vi "Sondenmodell.WriteZustandsgrössen.vi"(8 "Error in":errorcluster, 9 "Rücklauftemperatur Solekreislauf [°C]":dbl, 10 "Erdtemperatur [°C]":dbl, 11 "Sondemodell in":refnum<data-value>) -> (0 "Error out":errorcluster)   [LabVIEW 2016, in "Sondenmodell.lvclass"]
uses:
  Sondenmodell.lvclass
  Sondenmodell.lvclass/Sondenmodell.ctl
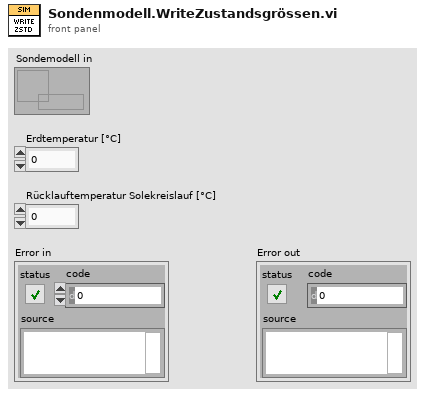
[diagram p1: front panel]
types:
  T1 = typedef "Sondenmodell.lvclass/Sondenmodell.Zustandsgrössen.ctl" = cluster{"Erdtemperatur [°C]":dbl, "Rücklauftemperatur Solekreislauf [°C]":dbl}
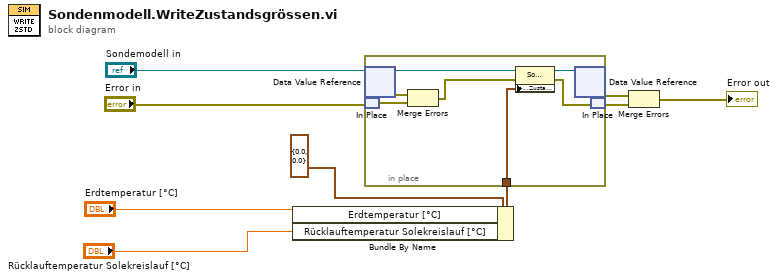
[diagram p0: block diagram]
diagram:
  n1 = Bundle By Name(cluster=T1 {"Erdtemperatur [°C]"=0.0, "Rücklauftemperatur Solekreislauf [°C]"=0.0} ("Sondenmodell.Zustandsgrössen"), "Erdtemperatur [°C]"="Erdtemperatur [°C]", "Rücklauftemperatur Solekreislauf [°C]"="Rücklauftemperatur Solekreislauf [°C]") -> (w5:T1)
  n2 = in-place {
    in-place-border: w5 -> [w10]
    n3 = in-place-dvr #1("Sondemodell in") -> (w16:refnum<class "Sondenmodell.lvclass">, w13:errorcluster)
    n4 = in-place-match #2("Error in") -> (w12:errorcluster)
    n5 = Merge Errors(w13, w12) -> (w14:errorcluster)
    n6 = property class="Sondenmodell.lvclass"(reference=w16, error in=w14, "Accessors:Sondenmodell.Zustandsgrössen"=w10) -> (reference out=w15:refnum<class "Sondenmodell.lvclass">, error out=w11:errorcluster)
    n7 = in-place-dvr #1(w15) -> (w8:errorcluster)  [unwired: 1 out]
    n8 = in-place-match #2(w11) -> (w7:errorcluster)
  }
  n9 = Merge Errors(w8, w7) -> (→"Error out":errorcluster)
